vi "hardware_close_hardware.vi"(8 "error in (no error)":errorcluster, 11 "thorlabs_FW102C in":refnum<class "thorlabs_FW102C.lvclass">) -> (0 "error out":errorcluster, 3 "thorlabs_FW102C out":refnum<class "thorlabs_FW102C.lvclass">)   [LabVIEW 2015, in "thorlabs_FW102C.lvclass"]
uses:
  thorlabs_FW102C.lvclass
  thorlabs_FW102C.lvclass/thorlabs_FW102C.ctl
  Thorlabs_FW102C.lvlib
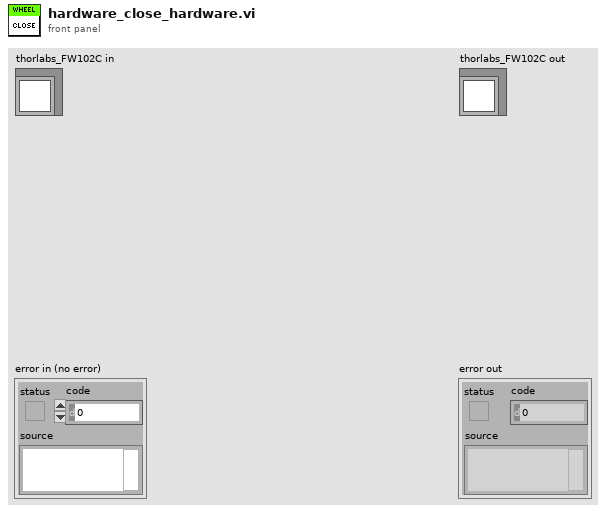
[diagram p1: front panel]
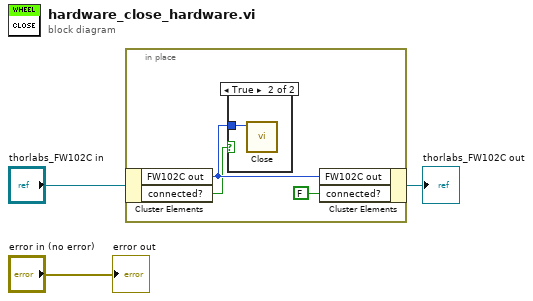
[diagram p0: block diagram]
diagram:
  n1 = in-place {
    n2 = in-place-cluster #1("thorlabs_FW102C in") -> ("FW102C out"=w6:i32, "connected?"=w5:bool)
    n3 = case shown="True" w5 {
      tunnel: w6 -> [_ w7]
      frame False {
      }
      frame True {
        n4 = call "Close.vi"("FW102C in"=w7) -> ()  [unwired: 10 in, 1 out]
      }
    }
    n5 = in-place-cluster #1("FW102C out"=w6, "connected?"=FALSE) -> (→"thorlabs_FW102C out":refnum<class "thorlabs_FW102C.lvclass">)
  }
  "error out" <- "error in (no error)"
